vi "Inquire Table.vi"(0 "表格":refnum<vi>, 11 "error in (no error)":errorcluster caption="错误输入（无错误）") -> (3 "Type":string, 4 "Num&Angle":dbl[][](array[numeric]), 6 "XY图/Num&Angle":cluster{dbl[], dbl[]}, 8 "选择的ID":string[](array[string]), 10 "选择的列首":string, 14 "Class&Num&Angle":dbl[][](array[numeric]), 15 "error out":errorcluster caption="错误输出")   [LabVIEW 2016]
panel:
  out "子数组":string[][](array[string])
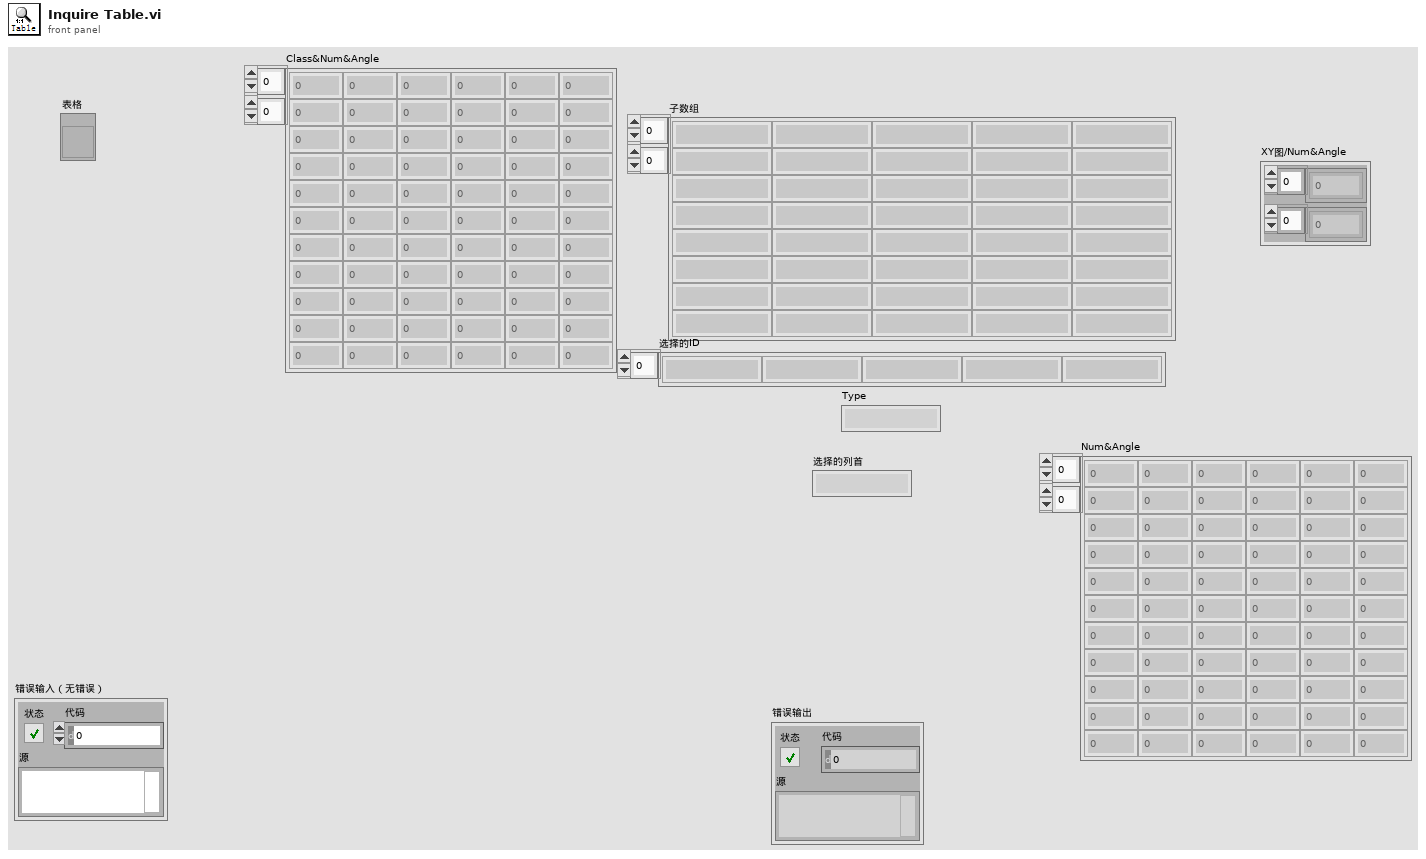
[diagram p1: front panel]
types:
  T1 = typedef "LVRowAndColumnTypeDef.ctl" = cluster{"Row":i32, "Column":i32}
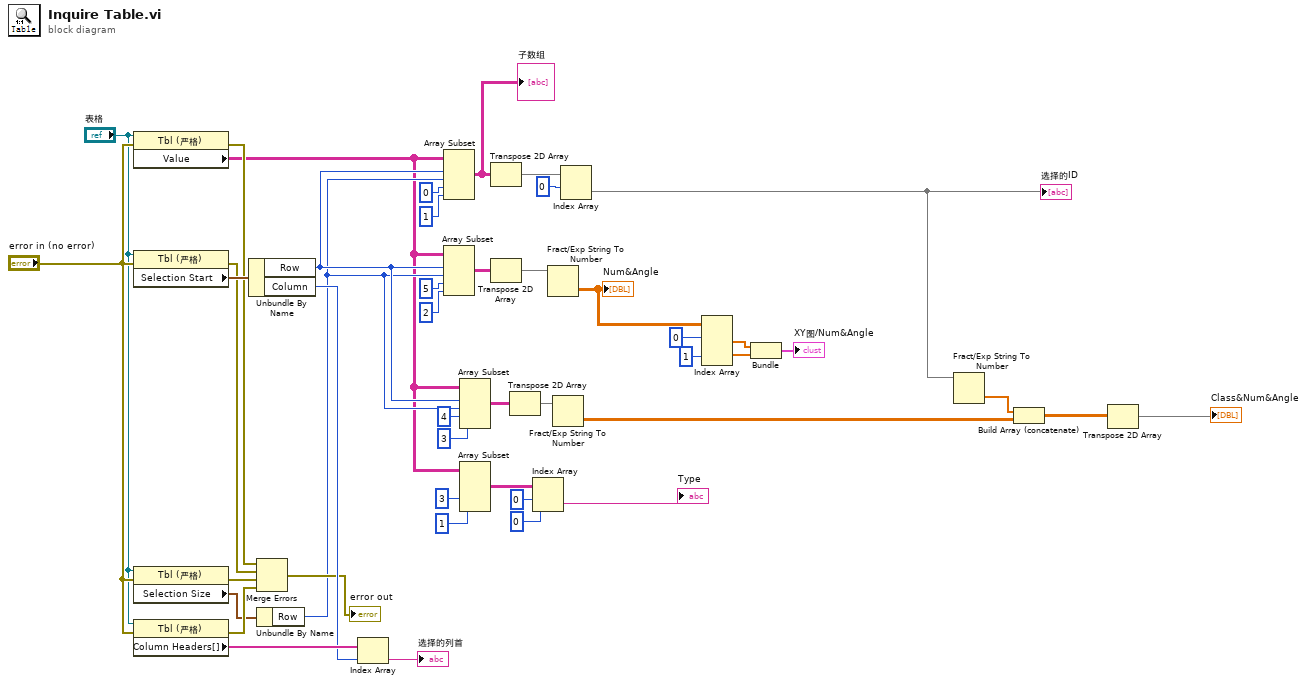
[diagram p0: block diagram]
diagram:
  n1 = property class="Tbl (严格)"(reference="表格", error in="error in (no error)") -> (error out=w35:errorcluster, "Value"=w9:string[][])  [unwired: 1 out]
  n2 = property class="Tbl (严格)"(reference="表格", error in="error in (no error)") -> (error out=w34:errorcluster, "Selection Start"=w45:T1)  [unwired: 1 out]
  n3 = property class="Tbl (严格)"(reference="表格", error in="error in (no error)") -> (error out=w33:errorcluster, "Selection Size"=w30:T1)  [unwired: 1 out]
  n4 = property class="Tbl (严格)"(reference="表格", error in="error in (no error)") -> (error out=w32:errorcluster, "Column Headers[]"=w38:string[])  [unwired: 1 out]
  n5 = Unbundle By Name(w45) -> ("Row"=w18:i32, "Column"=w37:i32)
  n6 = Merge Errors(w35, w34, w33, w32) -> (→"error out":errorcluster)
  n7 = Unbundle By Name(w30) -> ("Row"=w17:i32)
  n8 = Index Array(array=w38, index=w37) -> (element=→"选择的列首":string)
  n9 = Array Subset(array=w9, index (row)=w18, length (row)=w17, index (col)=0 ("索引"), length (col)=1 ("长度")) -> (w42:string[][])
  "子数组" <- w42
  n10 = Array Subset(array=w9, index (row)=w18, length (row)=w17, index (col)=5 ("索引"), length (col)=2 ("长度")) -> (w26:string[][])
  n11 = Array Subset(array=w9, index (row)=w18, length (row)=w17, index (col)=4 ("索引"), length (col)=3 ("长度")) -> (w14:string[][])
  n12 = Array Subset(array=w9, index (col)=3 ("索引"), length (col)=1 ("长度")) -> (w6:string[][])  [unwired: 2 in]
  n13 = Transpose 2D Array(2D array=w42) -> (transposed array=w41:string[][])
  n14 = Transpose 2D Array(2D array=w26) -> (transposed array=w25:string[][])
  n15 = Transpose 2D Array(2D array=w14) -> (transposed array=w13:string[][])
  n16 = Index Array(array=w6, index (row)=0 ("索引 (行)"), index (col)=0 ("禁用的索引 (列)")) -> (element=→"Type":string)
  n17 = Fract/Exp String To Number(string=w25) -> (number=w20:dbl[][])  [unwired: 3 in, 1 out]
  "Num&Angle" <- w20
  n18 = Fract/Exp String To Number(string=w13) -> (number=w10:dbl[][])  [unwired: 3 in, 1 out]
  n19 = Index Array(array=w41, index (row)=0 ("索引 (行)")) -> (element=w12:string[])  [unwired: 1 in]
  "选择的ID" <- w12
  n20 = Index Array(array=w20, index (row) #1=0 ("索引 (行)"), index (row) #2=1 ("索引 (行)")) -> (element #1=w23:dbl[], element #2=w21:dbl[])  [unwired: 2 in]
  n21 = Bundle(w23, w21) -> (→"XY图/Num&Angle":cluster{dbl[], dbl[]})  [unwired: 1 in]
  n22 = Fract/Exp String To Number(string=w12) -> (number=w11:dbl[])  [unwired: 3 in, 1 out]
  n23 = Build Array (concatenate)(w11, w10) -> (w2:dbl[][])
  n24 = Transpose 2D Array(2D array=w2) -> (transposed array=→"Class&Num&Angle":dbl[][])
